vi "MDPtr SetStrAttribute.vi"(8 "String Attribute":string, 9 "error in (no error)":errorcluster, 10 "HexStrPtr":T1) -> (2 "error out":errorcluster, 3 "HexStrPtr (dup)":T1)   [LabVIEW 2017, in "MDPtr.lvlib"]
uses:
  MDPtr.lvlib
  MDPtr TypeDef/MDPtr.ctl
  MDPtr TypeDef/MDPtr DataFrame-PlaceHolder.ctl
  MDPtr TypeDef/MDPtr DataFrame-Common.ctl
  <vilib>/Utility/Data Type/Type Definitions/Data Type.ctl
  _Support/_MDPtr Build Error Cluster.vi
  <vilib>/Utility/Data Type/NI_Data Type.lvlib
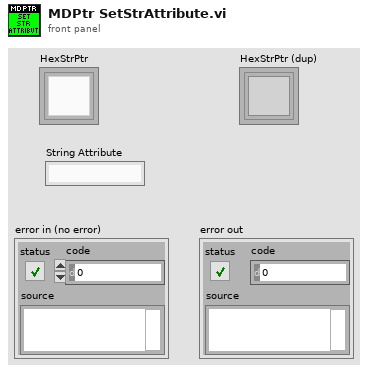
[diagram p1: front panel]
types:
  T1 = typedef "MDPtr.lvlib/MDPtr.ctl" = refnum<k1>
  T2 = typedef "MDPtr.lvlib/MDPtr DataFrame-PlaceHolder.ctl" = cluster{"Common":T3, "DVR":refnum<data-value>}
  T3 = typedef "MDPtr.lvlib/MDPtr DataFrame-Common.ctl" = cluster{"Data Type":T4, "Copy Count":i32, "String Attribute":string, "Cache Length":i32, "Data Length":i32}
  T4 = typedef "NI_Data Type.lvlib/Data Type.ctl" = enum8{"Invalid Type", "Void", "I8", "I16", "I32", "I64", "U8", "U16", "U32", "U64", "Single Float", "Double Float", "Extended Float", "Single Complex", "Double Complex", "Extended Complex", "Enum U8", "Enum U16", "Enum U32", "Enum U64", "Single Float With Unit", "Double Float With Unit", "Extended Float With Unit", "Single Complex with Unit", "Double Complex with Unit", "Extended Complex with Unit", "Boolean", "String", "Path", "Picture", "Tag", "Array", "Cluster", "Variant", "LV Variant", "Waveform", "Timestamp", "Digital Waveform", "Digital Data", "ExpressData", "Refnum", "External Data", "VI", "Poly VI", "LabVIEW Class Instance", "Fixed Point"}
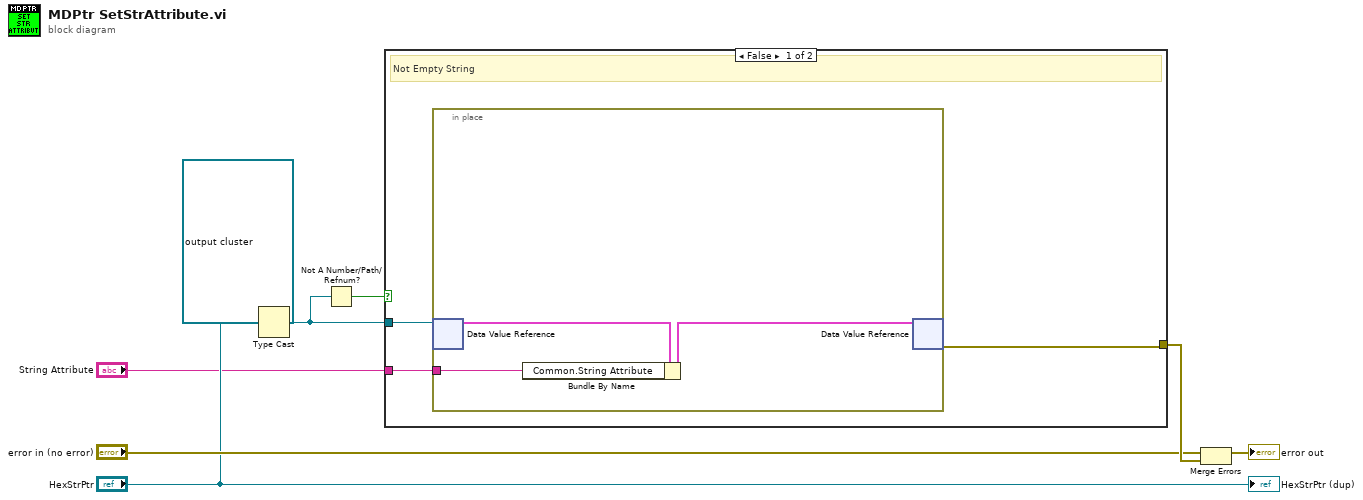
[diagram p0: block diagram]
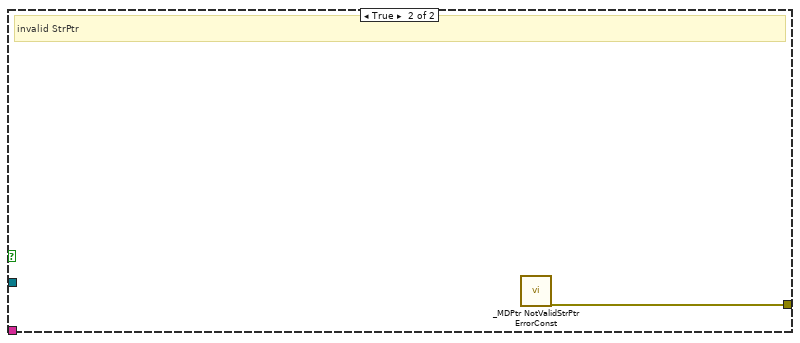
[diagram p2: hidden frame]
diagram:
  n1 = Type Cast(type=refnum<data-value> refnum ("data value reference"), x="HexStrPtr") -> (*(type *) &x=w2:refnum<data-value>)
  n2 = Not A Number/Path/Refnum?(number/path/refnum=w2) -> (NaN/Path/Refnum?=w3:bool)
  n3 = case shown="False" w3 {
    tunnel: [w9 w15] -> w8
    tunnel: w2 -> [w11 _]
    tunnel: "String Attribute" -> [w10 _]
    frame False {
      # "Not Empty String"
      n4 = in-place {
        in-place-border: w10 -> [w12]
        n5 = in-place-dvr #1(w11) -> (w14:T2)  [unwired: 1 out]
        n6 = Bundle By Name(cluster=w14, "Common.String Attribute"=w12) -> (w13:T2)
        n7 = in-place-dvr #1(w13) -> (w9:errorcluster)  [unwired: 1 out]
      }
    }
    frame True {
      # "invalid StrPtr"
      n8 = call "_MDPtr NotValidStrPtr ErrorConst.vi"() -> ("error out"=w15:errorcluster)  [unwired: 19 in]
    }
  }
  n9 = Merge Errors("error in (no error)", w8) -> (→"error out":errorcluster)
  "HexStrPtr (dup)" <- "HexStrPtr"
